vi "ValuesGotOverwrittenCalculator.vi"(1 "StrTableSize":i32, 2 "NumTableSize":i32, 3 "BoolTableSize":i32, 4 "disconnected":bool) -> (0 "ValuesGotOverwritten":bool)   [LabVIEW 2019]
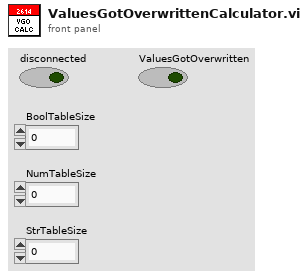
[diagram p1: front panel]
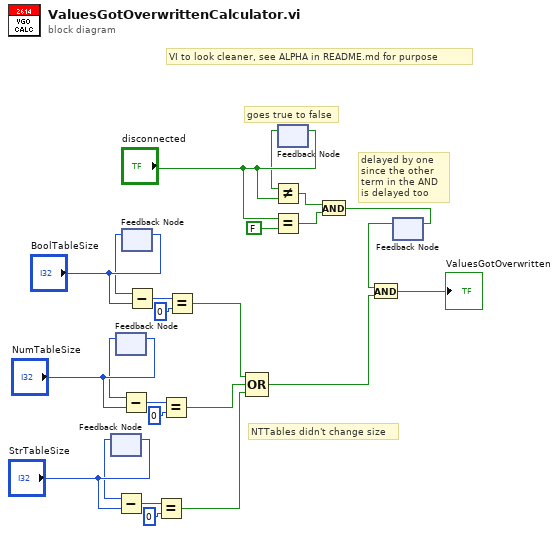
[diagram p0: block diagram]
diagram:
  # "VI to look cleaner, see ALPHA in README.md for purpose"
  # "NTTables didn't change size"
  # "delayed by one since the other term in the AND is delayed too"
  # "goes true to false"
  n1 = feedback #1() -> (w12:i32)  [unwired: 1 in]
  n2 = feedback-in #1("StrTableSize") -> ()
  n3 = feedback #2() -> (w11:i32)  [unwired: 1 in]
  n4 = feedback-in #2("NumTableSize") -> ()
  n5 = Subtract(x=w12, y="StrTableSize") -> (x-y=w13:i32)
  n6 = Subtract(x=w11, y="NumTableSize") -> (x-y=w10:i32)
  n7 = feedback #3() -> (w1:i32)  [unwired: 1 in]
  n8 = feedback-in #3("BoolTableSize") -> ()
  n9 = Subtract(x=w1, y="BoolTableSize") -> (x-y=w3:i32)
  n10 = Equal?(x=w13, y=0) -> (x = y?=w19:bool)
  n11 = Equal?(x=w10, y=0) -> (x = y?=w18:bool)
  n12 = Equal?(x=w3, y=0) -> (x = y?=w17:bool)
  n13 = Compound Arithmetic op=OR(w17, w18, w19) -> (w21:bool)
  n14 = Equal?(x="disconnected", y=FALSE) -> (x = y?=w8:bool)
  n15 = feedback #4() -> (w5:bool)  [unwired: 1 in]
  n16 = Not Equal?(x=w5, y="disconnected") -> (x != y?=w7:bool)
  n17 = feedback-in #4("disconnected") -> ()
  n18 = And(x=w7, y=w8) -> (x .and. y?=w24:bool)
  n19 = feedback #5() -> (w23:bool)  [unwired: 1 in]
  n20 = And(x=w23, y=w21) -> (x .and. y?=→"ValuesGotOverwritten":bool)
  n21 = feedback-in #5(w24) -> ()
